vi "Create Insertion Palette.vi"(8 "error in (no error)":errorcluster, 10 "Subpanel":refnum<vi>, 11 "TSnax UI Manager in":refnum<class "TSnax UI Manager.lvclass">) -> (0 "error out":errorcluster, 2 "Insertion Palette":refnum<class "InsertionPalettePanel.lvclass">, 3 "TSnax UI Manager out":refnum<class "TSnax UI Manager.lvclass">)   [LabVIEW 2020, in "TSnax UI.lvlib" / "TSnax UI Manager.lvclass"]
uses:
  TSnax UI Manager.lvclass
  TSnax UI Manager.lvclass/TSnax UI Manager.ctl
  <vilib>/IlluminatedG/IG OOPanel/OOPanel/Manager/Manager.lvclass
  InsertionPalettePanel/InsertionPalettePanel.lvclass
  C:/Program Files (x86)/National Instruments/LabVIEW 2020/vi.lib/IlluminatedG/IG OOPanel/OOPanel/Panel/Panel.lvclass
  C:/dev/illuminated-g/tsnax/TSnax UI/InsertionPalettePanel/InsertionPalettePanel.lvclass
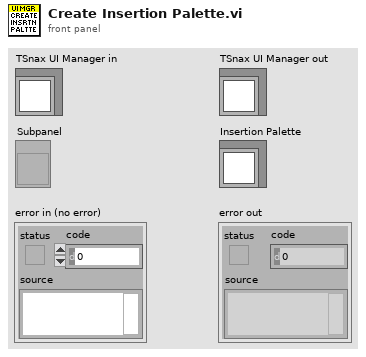
[diagram p1: front panel]
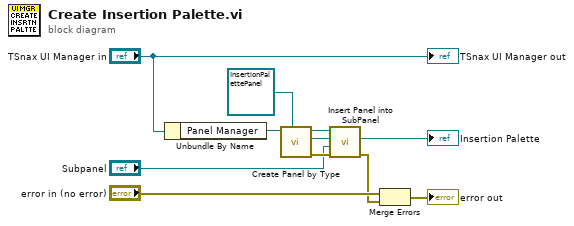
[diagram p0: block diagram]
diagram:
  n1 = Unbundle By Name("TSnax UI Manager in") -> ("Panel Manager"=w9:refnum<class "Manager.lvclass">)
  n2 = call <vilib>:"Create Panel by Type.vi"("Panel Type"=refnum<class "InsertionPalettePanel.lvclass"> refnum ("TSnax UI.lvlib:InsertionPalettePanel.lvclass"), "Manager in"=w9) -> ("error out"=w5:errorcluster, "Panel"=w6:refnum<class "InsertionPalettePanel.lvclass">, "Manager out"=w7:refnum<class "Manager.lvclass">)  [unwired: 7 in]
  n3 = call <vilib>:"Insert Panel into SubPanel.vi"("error in (no error)"=w5, "SubPanel"="Subpanel", "Panel In"=w6, "Manager in"=w7) -> ("error out"=w1:errorcluster, "Panel"=→"Insertion Palette":refnum<class "InsertionPalettePanel.lvclass">)  [unwired: 5 in, 1 out]
  n4 = Merge Errors("error in (no error)", w1) -> (→"error out":errorcluster)
  "TSnax UI Manager out" <- "TSnax UI Manager in"
